vi "Set Bit Value - U16.vi"(6 "BitValue":bool, 7 "BitPosition":T1, 10 "Data In":u16 format="%016b") -> (2 "Data Out":u16 format="%016b")   [LabVIEW 2012]
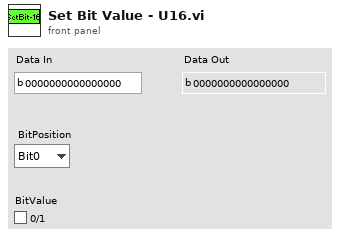
[diagram p1: front panel]
types:
  T1 = typedef "BitPosition(U16)" = enum16{"Bit0", "Bit1", "Bit2", "Bit3", "Bit4", "Bit5", "Bit6", "Bit7", "Bit8", "Bit9", "Bit10", "Bit11", "Bit12", "Bit13", "Bit14", "Bit15"}
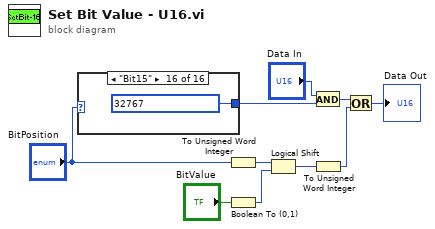
[diagram p0: block diagram]
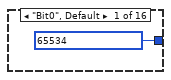
[diagram p2: hidden frame]
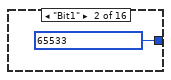
[diagram p3: hidden frame]
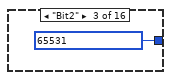
[diagram p4: hidden frame]
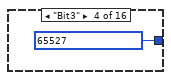
[diagram p5: hidden frame]
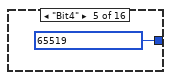
[diagram p6: hidden frame]
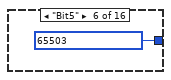
[diagram p7: hidden frame]
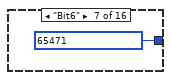
[diagram p8: hidden frame]
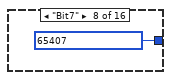
[diagram p9: hidden frame]
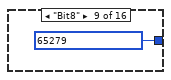
[diagram p10: hidden frame]
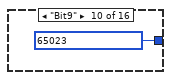
[diagram p11: hidden frame]
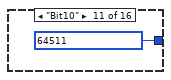
[diagram p12: hidden frame]
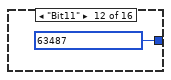
[diagram p13: hidden frame]
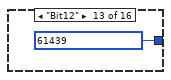
[diagram p14: hidden frame]
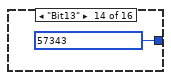
[diagram p15: hidden frame]
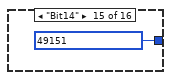
[diagram p16: hidden frame]
diagram:
  n1 = case shown="\"Bit15\"" "BitPosition" {
    tunnel: [u16 65534 ("Data") u16 65533 ("Data") u16 65531 ("Data") u16 65527 ("Data") u16 65519 ("Data") u16 65503 ("Data") u16 65471 ("Data") u16 65407 ("Data") u16 65279 ("Data") u16 65023 ("Data") u16 64511 ("Data") u16 63487 ("Data") u16 61439 ("Data") u16 57343 ("Data") u16 49151 ("Data") u16 32767 ("Data")] -> w9
    frame "Bit0", Default {
    }
    frame "Bit1" {
    }
    frame "Bit2" {
    }
    frame "Bit3" {
    }
    frame "Bit4" {
    }
    frame "Bit5" {
    }
    frame "Bit6" {
    }
    frame "Bit7" {
    }
    frame "Bit8" {
    }
    frame "Bit9" {
    }
    frame "Bit10" {
    }
    frame "Bit11" {
    }
    frame "Bit12" {
    }
    frame "Bit13" {
    }
    frame "Bit14" {
    }
    frame "Bit15" {
    }
  }
  n2 = To Unsigned Word Integer(number="BitPosition") -> (unsigned 16bit integer=w7:u16)
  n3 = Boolean To (0,1)(Boolean="BitValue") -> (0, 1=w5:i16)
  n4 = Logical Shift(y=w7, x=w5) -> (x << y=w3:i16)
  n5 = And(x="Data In", y=w9) -> (x .and. y?=w8:u16)
  n6 = To Unsigned Word Integer(number=w3) -> (unsigned 16bit integer=w1:u16)
  n7 = Or(x=w8, y=w1) -> (x .or. y?=→"Data Out":u16)
